vi "Remove small insects.vi"(1 "2D array with insects data":dbl[][](array[numeric]), 2 "Max size of insects":dbl) -> (0 "2D array (smaller insects removed)":dbl[][](array[numeric]))   [LabVIEW 2022 SP3]
doc: "Removes insects smaller specified"
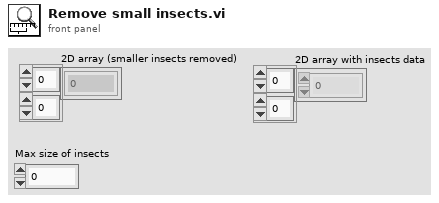
[diagram p1: front panel]
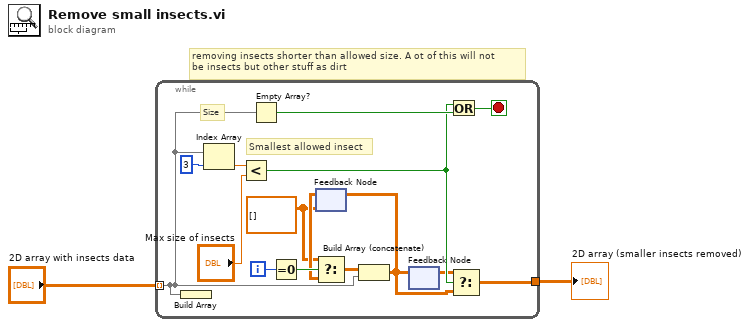
[diagram p0: block diagram]
diagram:
  # "removing insects shorter than allowed size. A ot of this will not \nbe insects but other stuff as dirt"
  n1 = while {
    tunnel: "2D array with insects data" -> [w4] mode=indexing
    tunnel: [w12] -> w2
    i -> [w9]
    stop <- w14 stop-if-true
    w5 = dbl[][] []
    # "Smallest allowed insect"
    # "Size"
    n2 = Build Array(w4) -> ()  [unwired: 1 out]
    n3 = Index Array(array=w4, index=3) -> (element=w16:dbl)
    n4 = Less?(x=w16, y="Max size of insects") -> (x < y?=w13:bool)
    n5 = Empty Array?(array=w4) -> (empty?=w15:bool)
    n6 = Equal To 0?(x=w9) -> (x = 0?=w8:bool)
    n7 = feedback #1(w5) -> (w6:dbl[][])
    n8 = Select(t=w5, s=w8, f=w6) -> (s? t:f=w7:dbl[][])
    n9 = Build Array (concatenate)(w7, w4) -> (w11:dbl[][])
    n10 = feedback-in #1(w11) -> ()
    n11 = feedback-in #2(w11) -> ()
    n12 = feedback #2() -> (w10:dbl[][])  [unwired: 1 in]
    n13 = Or(x=w13, y=w15) -> (x .or. y?=w14:bool)
    n14 = Select(t=w10, s=w13, f=w11) -> (s? t:f=w12:dbl[][])
  }
  "2D array (smaller insects removed)" <- w2
